vi "Pre Launch Init.vi"(11 "Device in":refnum<class "Device.lvclass">) -> (0 "error out":errorcluster, 3 "Device out":refnum<class "Device.lvclass">)   [LabVIEW 2014, in "DAQ Device.lvlib" / "Device.lvclass"]
doc: "(<B>Filename</B>: Actor Framework.lvlib:Actor.lvclass:Pre Launch Init.vi)\n\nDefines behavior that occurs after the Launch Nested Actor method is invoked but before the actor's Actor Core method begins running.\n\nBy default, this method does nothing. A descendant class may override it to define behavior."
uses:
  Device.lvclass
  SuperActor/Ex Nested.lvclass
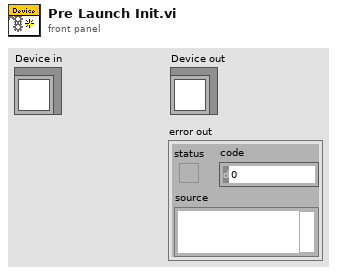
[diagram p1: front panel]
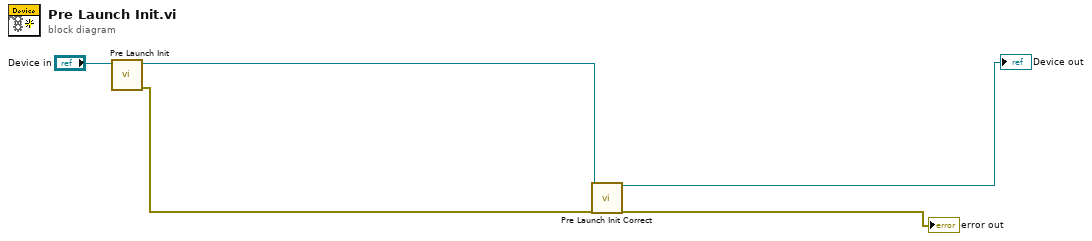
[diagram p0: block diagram]
diagram:
  n1 = call-parent "Pre Launch Init.vi"("Ex Nested in"="Device in") -> ("error out"=w1:errorcluster, "Ex Nested out"=w2:refnum<class "Device.lvclass">)  [unwired: 9 in]
  n2 = call "Pre Launch Init Correct.vi"("Device in"=w2, "error in (no error)"=w1) -> ("Device out"=→"Device out":refnum<class "Device.lvclass">, "error out"=→"error out":errorcluster)  [unwired: 16 in]
